vi "Start Vecto.vi"(8 "error in (no error)":errorcluster, 11 "Volatus Core in":refnum<class "Volatus Core.lvclass">) -> (0 "error out":errorcluster, 3 "Volatus Core out":refnum<class "Volatus Core.lvclass">)   [LabVIEW 2020, in "Volatus.lvlib" / "Volatus Core.lvclass"]
uses:
  Volatus Core.lvclass
  Volatus Core.lvclass/Volatus Core.ctl
  lv-vecto/Vecto/Vecto/Vecto.lvclass
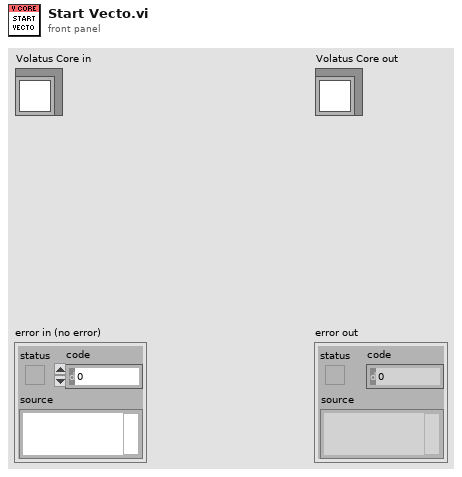
[diagram p1: front panel]
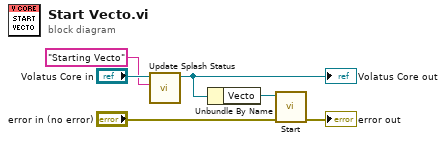
[diagram p0: block diagram]
diagram:
  n1 = call "Update Splash Status.vi"("Status"="Starting Vecto", "Volatus Core in"="Volatus Core in") -> ("Volatus Core out"=w2:refnum<class "Volatus Core.lvclass">)  [unwired: 8 in, 1 out]
  "Volatus Core out" <- w2
  n2 = Unbundle By Name(w2) -> ("Vecto"=w5:refnum<class "Vecto.lvclass">)
  n3 = call "Start.vi"("error in (no error)"="error in (no error)", "Vecto in"=w5) -> ("error out"=→"error out":errorcluster)  [unwired: 8 in, 1 out]
